vi "Dependency.vi"() -> ()   [LabVIEW 2020, in "Dependency.lvlib"]
uses:
  Dependency.lvlib
panel:
  out "its working!":bool=TRUE
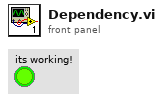
[diagram p1: front panel]
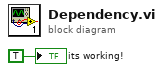
[diagram p0: block diagram]
diagram:
  "its working!" <- TRUE
